vi "Diagnostics - Tool.vi"() -> ()   [LabVIEW 2015, in "Diagnostics Tool.lvlib"]
uses:
  Diagnostics Tool.lvlib
  Shared/Types/Command.ctl
  NationalInstruments.VeriStand.SystemStorage
  Shared/Types/Workspace.State.ctl
  Shared/Types/UI.Refs.ctl
  <vilib>/NI Veristand/Display Template Support/Display Template Support.llb/enum_Display Template Handler Minimal To Workspace.ctl
  Shared/Types/Workspace.SavedState.ctl
  <vilib>/NI Veristand/Execution/Workspace/WorkspaceAPI.ctl
  <vilib>/NI Veristand/Display Template Support/Display Template Support.llb/enum_Display Template Handler Minimal To Widget Msg.ctl
  <vilib>/NI Veristand/Execution/Workspace/SystemStateRegEventRef.ctl
  <vilib>/NI Veristand/Execution/Workspace/Target State Info.ctl
  <vilib>/NI Veristand/Execution/Workspace/Target State.ctl
  <vilib>/NI Veristand/Execution/Workspace/SystemStateEventRef.ctl
  Shared/Types/Protocol.ctl
  Shared/Types/Command.ReadDTC.ctl
  Shared/SubVIs/Constants.vi
  <vilib>/NI Veristand/Execution/Workspace/NI VeriStand - Get Multiple Channel Values.vi
  <vilib>/NI Veristand/Execution/Workspace/NI VeriStand - Set Multiple Channel Values.vi
  Shared/Diagnostics Addon Shared.lvlib
  <vilib>/NI Veristand/Execution/Workspace/NI_VS Workspace ExecutionAPI.lvlib
  Automation API/Diagnostics Host Automation API.lvlib
  NationalInstruments.VeriStand.ClientAPI
panel:
  out "Control Name":string
  in  "Tab Control":enum32{"Cmd", "Raw (TCP)", "Read DTCs (TCP)"}(tab)
  in  "Send":bool
  out "Data Length":i64
  out "VeriStand Error":i64 format="%.0x"
  out "Error Byte":i64 format="%.0x"
  out "Success?":bool
  in  "MetaData1":i64 format="%.0x"
  in  "MetaData2":i64 format="%.0x"
  in  "MetaData3":i64 format="%.0x"
  in  "MetaData4":i64 format="%.0x"
  in  "Cmd":T1
  in  "Clear":bool
  out "VeriStand Error":errorcluster
  out "Error Byte":u8 format="%.0x"
  in  "Response Required?":bool
  in  "Send Raw":bool
  out "Raw Resp":u8[](array[numeric]) format="%.0x"
  in  "Raw Cmd":u8[](array[numeric]) format="%.0x"
  in  "Extension":u32 format="%.0x"
  in  "Mask":u32 format="%.0x"
  in  "Mode":u32 format="%.0x"
  in  "Hex":bool
  in  "DTCs":i32(listbox)
  in  "Read DTCs":bool
  in  "NIVS.Gateway IP Address":string
  in  "NIVS.System Definition Root":refnum<k24>
  in  "NIVS.Workspace Event":refnum<event-registration>
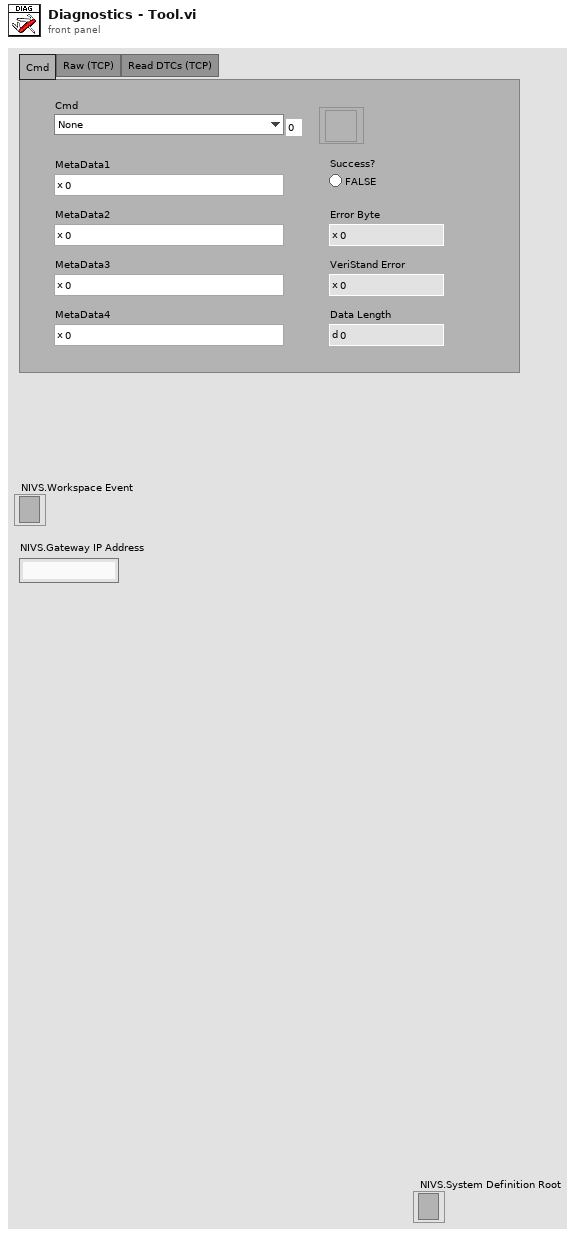
[diagram p1: front panel]
types:
  T1 = typedef "Diagnostics Addon Shared.lvlib/Command.ctl" = enum8{"None", "EnableDiagnosticSession", "DisableDiagnosticSession", "ReadDataIdentifiers", "ReadDataIdentifier", "WriteDataIndentifier", "ReadPIDsOnDemand", "ReadPIDOnDemand", "WriteCPID", "WriteMemory", "ReadMemory", "ReadDTCs", "ClearDTCs", "ControlDTC", "ForceTesterPresent", "DisableNormalCommunication", "ReturnToNormalMode", "InputOutputControl", "StartRoutine", "RequestRoutineStatus", "StopRoutine", "ECUReset", "UnlockECU", "ClearSuccessBit", "ConfigureandStartPIDs", "StopPIDs", "StartDTCs", "EnableChangeDTCCount", "DisableChangeDTCCount", "ReadFailureRecordParameters", "PassThru Channel Based", "EnableRepeatingTesterPresent", "DisableRepeatingTesterPresent"}
  T2 = typedef "Diagnostics Addon Shared.lvlib/Workspace.State.ctl" = cluster{"UI.Refs":T3, "Data.PreviousValues":dbl[], "Data.Read":string[], "CachedData.UserEvent":refnum<user-event>, "CachedData":T4, "Workspace.Connected?":bool, "NIVS.SysDef":refnum<k24>, "NIVS.WorkspaceManager":T5, "NIVS.UserEventRefs":cluster{"Event Registration Refnum":refnum<event-registration>, "SystemChangeEventRef":T6, "NIVS.Workspace Event":refnum<event-registration>}, "NIVS.SystemStateRefs":T7, "NIVS.LaunchRef":refnum<user-event>, "Data.PendingChange?":bool, "Data.Write":string[], "Diagnostic Protocol":T8, "Channels.Found":bool}
  T3 = typedef "Diagnostics Addon Shared.lvlib/UI.Refs.ctl" = cluster{"Cmd":refnum<vi>, "MetaData1":refnum<vi>, "MetaData2":refnum<vi>, "MetaData3":refnum<vi>, "MetaData4":refnum<vi>, "Success?":refnum<vi>, "ErrorByte":refnum<vi>, "VeriStandError":refnum<vi>, "DataLength":refnum<vi>}
  T4 = typedef "Diagnostics Addon Shared.lvlib/Workspace.SavedState.ctl" = cluster{"CD Path":string, "CD IP":string}
  T5 = typedef "NI_VS Workspace ExecutionAPI.lvlib/WorkspaceAPI.ctl" = refnum<k24>
  T6 = typedef "NI_VS Workspace ExecutionAPI.lvlib/SystemStateRegEventRef.ctl" = refnum<event-registration>
  T7 = typedef "NI_VS Workspace ExecutionAPI.lvlib/SystemStateEventRef.ctl" = cluster{"CustDatRef":refnum<user-event>, "EvtRef":refnum<k27>, "Target State User Event":refnum<user-event>}
  T8 = typedef "Diagnostics Addon Shared.lvlib/Protocol.ctl" = enum16{"GMLAN", "KWP-2000", "UDS", "User-Defined"}
  T9 = typedef "enum_Display Template Handler Minimal To Workspace.ctl" = cluster{"Operation":enum16{"SetCustomData", "DeleteItem"}, "Data":variant}
  T10 = typedef "Diagnostics Addon Shared.lvlib/Command.ReadDTC.ctl" = cluster{"Extension":u32, "Mask":u32, "Mode":u32}
  T11 = cluster{"Event Registration Refnum":refnum<event-registration>, "SystemChangeEventRef":T6, "NIVS.Workspace Event":refnum<event-registration>}
  T12 = typedef "NI_VS Workspace ExecutionAPI.lvlib/SystemState.ctl" = u8
  T13 = typedef "enum_Display Template Handler Minimal To Widget Msg.ctl" = enum16{"Stop", "LaunchConfigDialog"}
  T14 = typedef "stm_TCP Connection Info.ctl" = cluster{"connection ID":refnum<k5>, "Meta data":T15[]}
  T15 = typedef "stm_MetaDataElement.ctl" = string
  T16 = cluster{"resp":u8[], "error code":u8, "error out":errorcluster}
  T17 = typedef "Diagnostics Addon Shared.lvlib/DTC.Info.ctl" = cluster{"Timestamp":dbl, "DTC":dbl, "Status":dbl, "Add Data":dbl}
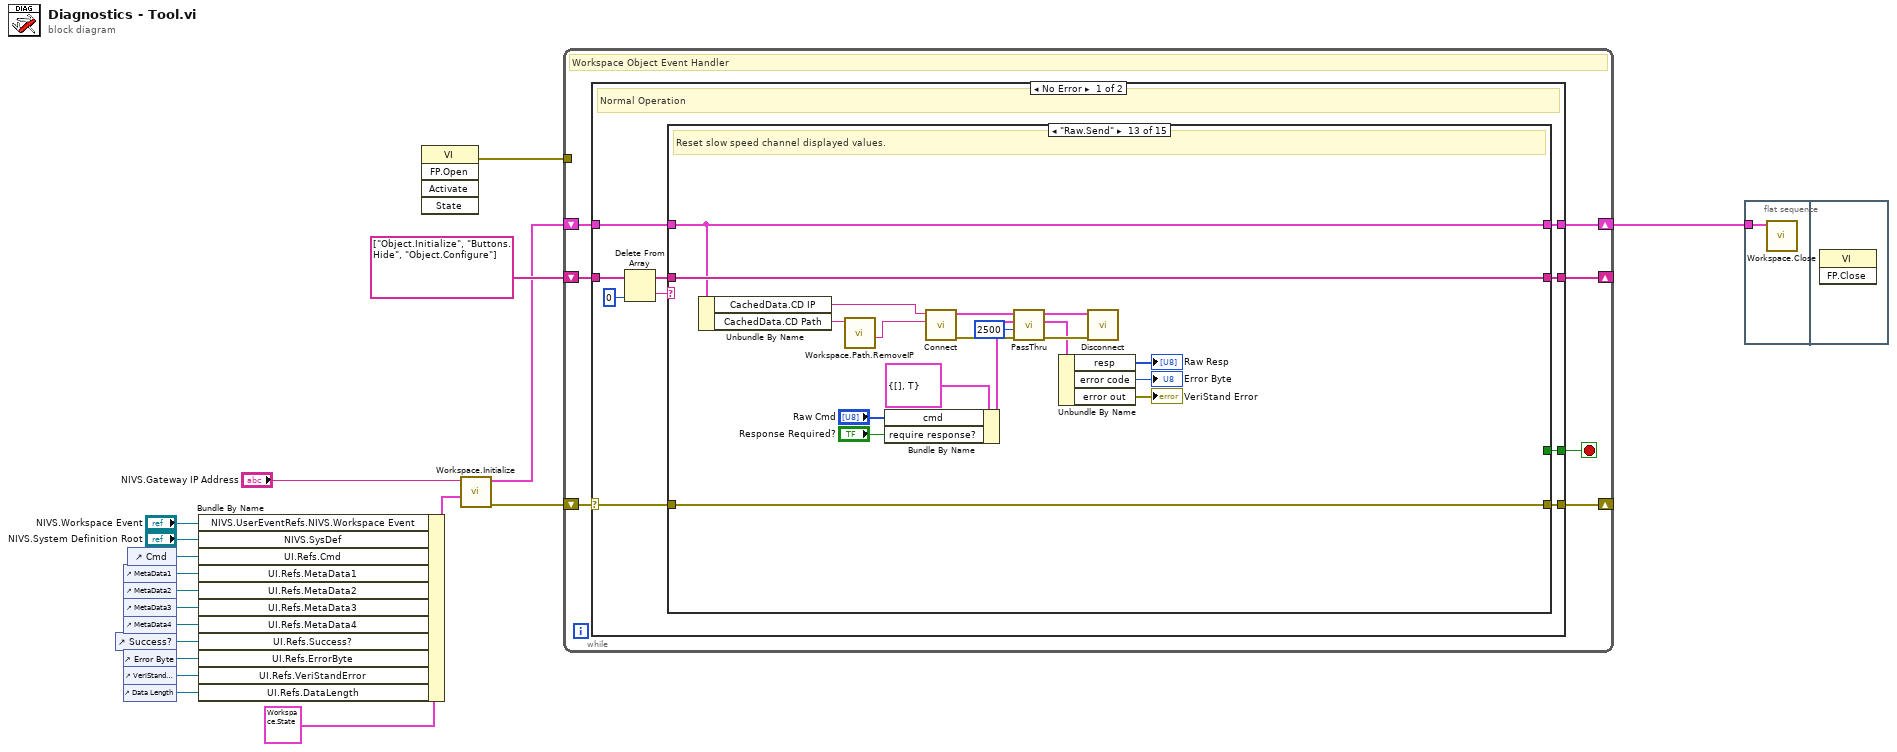
[diagram p0: block diagram]
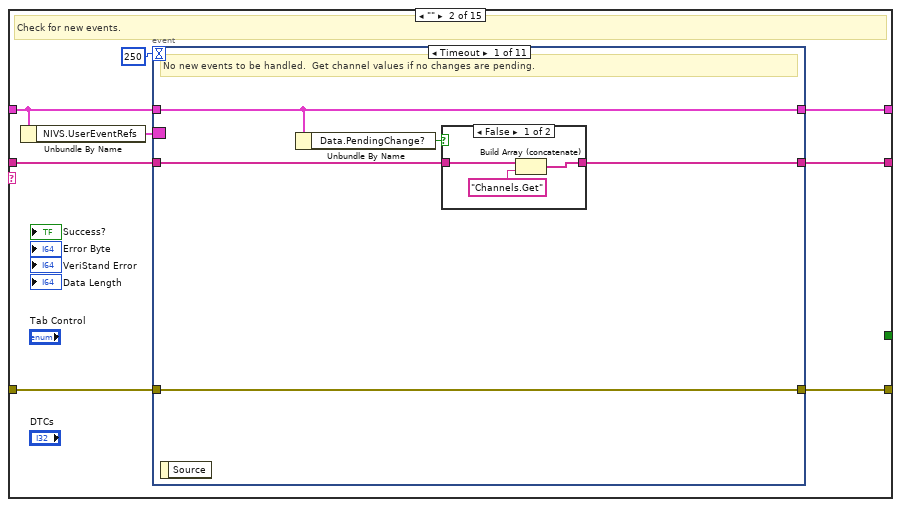
[diagram p3: hidden frame]
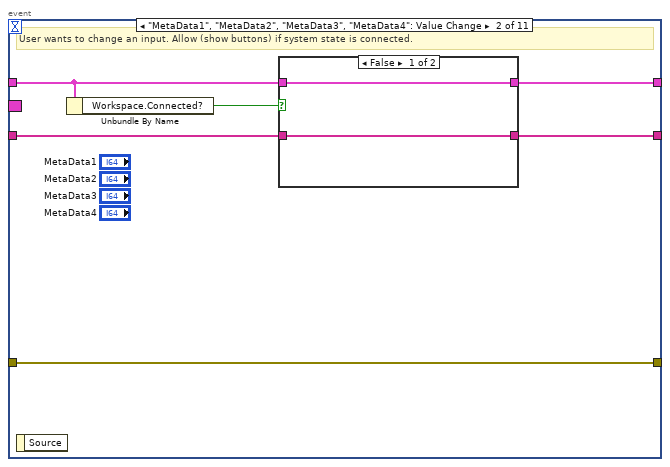
[diagram p5: hidden frame]
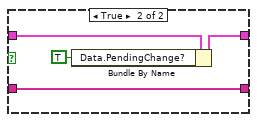
[diagram p6: hidden frame]
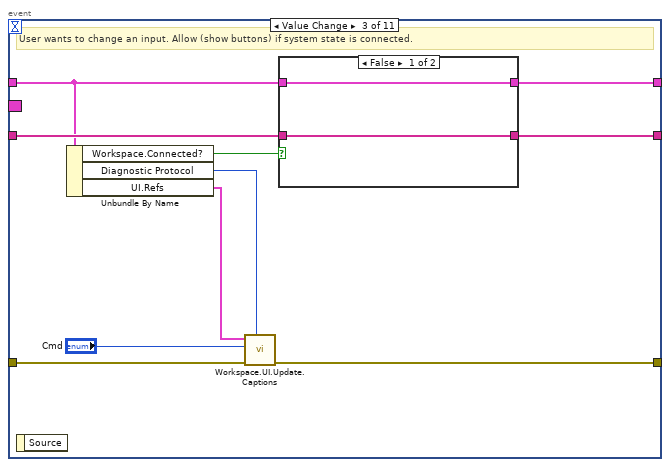
[diagram p7: hidden frame]
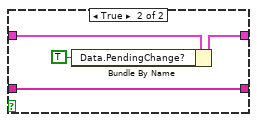
[diagram p8: hidden frame]
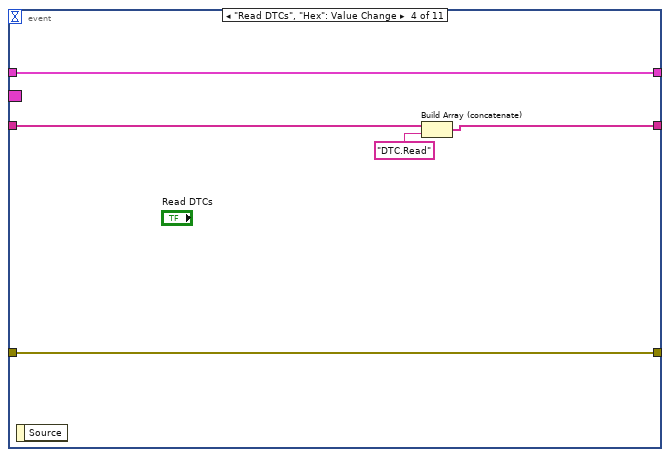
[diagram p9: hidden frame]
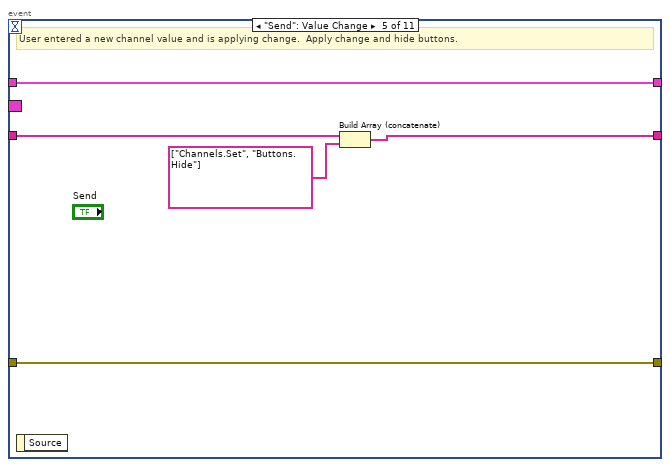
[diagram p10: hidden frame]
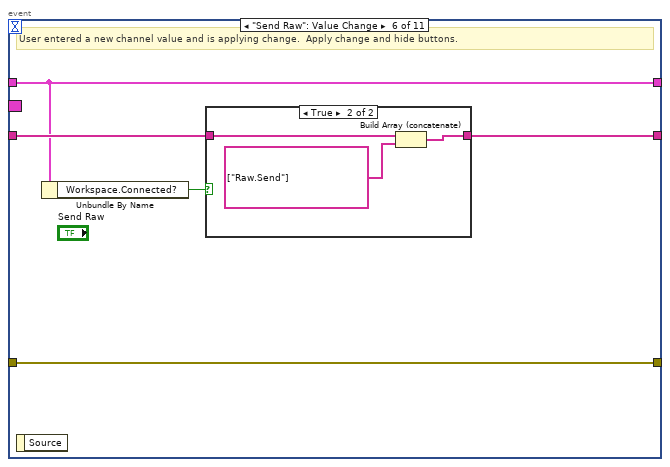
[diagram p11: hidden frame]
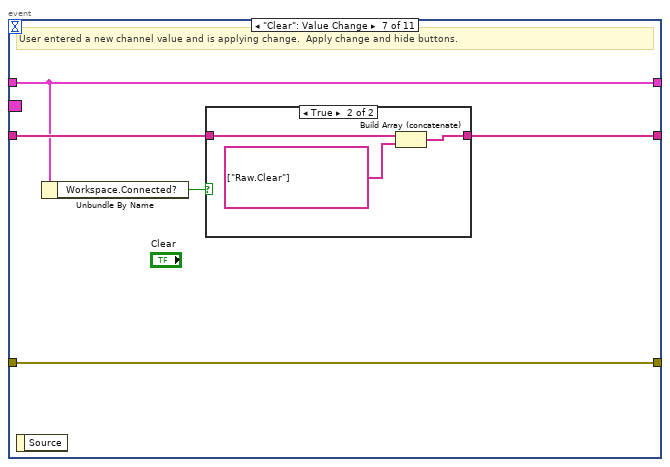
[diagram p13: hidden frame]
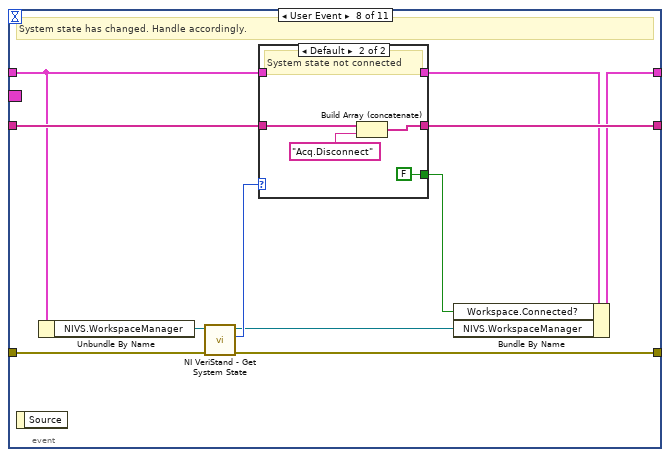
[diagram p15: hidden frame]
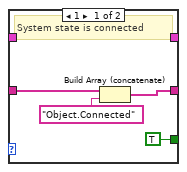
[diagram p16: hidden frame]
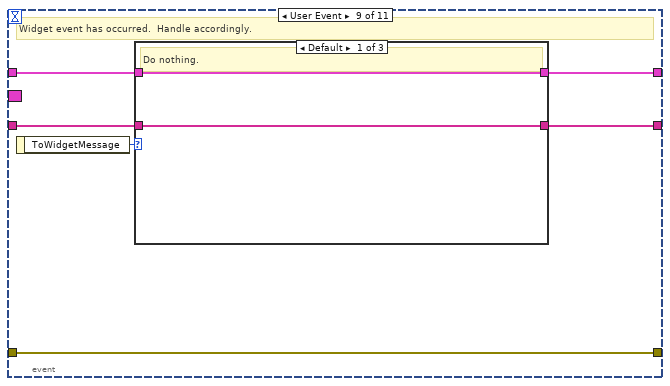
[diagram p17: hidden frame]
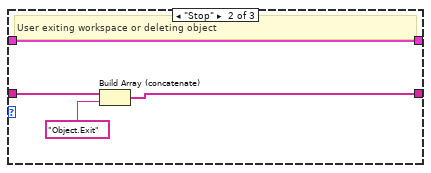
[diagram p18: hidden frame]
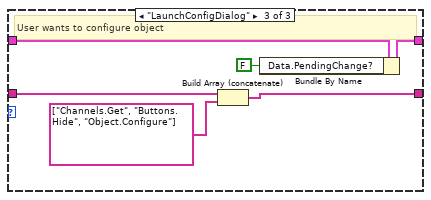
[diagram p19: hidden frame]
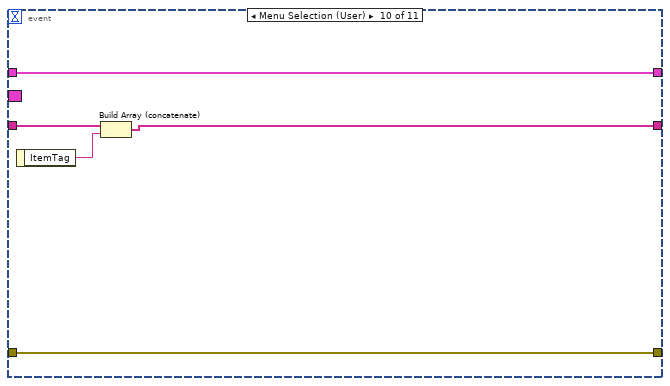
[diagram p20: hidden frame]
diagram:
  n1 = control-ref of="Success?"() -> (w4:refnum<vi>)
  n2 = control-ref of="MetaData1"() -> (w8:refnum<vi>)
  n3 = control-ref of="MetaData2"() -> (w7:refnum<vi>)
  n4 = control-ref of="MetaData3"() -> (w6:refnum<vi>)
  n5 = control-ref of="MetaData4"() -> (w5:refnum<vi>)
  n6 = control-ref of="Error Byte"() -> (w3:refnum<vi>)
  n7 = control-ref of="VeriStand Error"() -> (w2:refnum<vi>)
  n8 = control-ref of="Data Length"() -> (w1:refnum<vi>)
  n9 = control-ref of="Cmd"() -> (w9:refnum<vi>)
  n10 = Bundle By Name(cluster=T2 {"UI.Refs"={"Cmd"=refnum, "MetaData1"=refnum, "MetaData2"=refnum, "MetaData3"=refnum, "MetaData4"=refnum, "Success?"=refnum, "ErrorByte"=refnum, "VeriStandError"=refnum, "DataLength"=refnum}, "Data.PreviousValues"=[], "Data.Read"=[], "CachedData.UserEvent"=refnum, "CachedData"={"CD Path"="", "CD IP"=""}, "Workspace.Connected?"=FALSE, "NIVS.SysDef"=refnum, "NIVS.WorkspaceManager"=refnum, "NIVS.UserEventRefs"={"Event Registration Refnum"=refnum, "SystemChangeEventRef"=refnum, "NIVS.Workspace Event"=refnum}, "NIVS.SystemStateRefs"={"CustDatRef"=refnum, "EvtRef"=refnum, "Target State User Event"=refnum}, "NIVS.LaunchRef"=refnum, "Data.PendingChange?"=FALSE, "Data.Write"=[], "Diagnostic Protocol"=enum."GMLAN", "Channels.Found"=FALSE}, "NIVS.UserEventRefs.NIVS.Workspace Event"="NIVS.Workspace Event", "NIVS.SysDef"="NIVS.System Definition Root", "UI.Refs.Cmd"=w9, "UI.Refs.MetaData1"=w8, "UI.Refs.MetaData2"=w7, "UI.Refs.MetaData3"=w6, "UI.Refs.MetaData4"=w5, "UI.Refs.Success?"=w4, "UI.Refs.ErrorByte"=w3, "UI.Refs.VeriStandError"=w2, "UI.Refs.DataLength"=w1) -> (w18:T2)
  n11 = invoke class="VI" method="FP.Open"() -> (error out=w11:errorcluster)  [unwired: 5 in, 4 out]
  n12 = call "Workspace.Initialize.vi"("State Variables in"=w18, "NIVS.Gateway IP Address"="NIVS.Gateway IP Address") -> ("error out"=w14:errorcluster, "State Variables out"=w12:T2)  [unwired: 8 in]
  n13 = while {
    shift-right: [w24] -> _
    shift-left: string[] ["Object.Initialize", "Buttons.Hide", "Object.Configure"] -> [w25]
    shift-right: [w22] -> w10
    shift-left: w12 -> [w21]
    shift-right: [w23] -> _
    shift-left: w14 -> [w20]
    tunnel: w11 -> [_]
    stop <- w26 stop-if-true
    # "Workspace Object Event Handler"
    n14 = case shown="No Error" w20 {
      selector: w20 -> [w27 w385]
      tunnel: [w36 _] -> w26
      tunnel: w25 -> [w34 w392]
      tunnel: [w31 w392] -> w24
      tunnel: [w30 w383] -> w23
      tunnel: [w29 w391] -> w22
      tunnel: w21 -> [w28 w391]
      frame No Error {
        # "Normal Operation"
        n15 = Delete From Array(array=w34, index=0) -> (deleted portion=w33:string, array with subset deleted=w32:string[])  [unwired: 1 in]
        n16 = case shown="\"Raw.Send\"" w33 {
          tunnel: [_ _ _ _ _ TRUE _ _ _ _ _ _ _ _ _] -> w36
          tunnel: [w39 w46 w182 w199 w230 w246 w253 w256 w259 w268 w301 w314 w333 w337 w358] -> w31
          tunnel: w27 -> [w38 w44 w183 w205 w227 w243 w252 w254 w257 w266 w300 w313 w332 w336 w346]
          tunnel: w32 -> [w39 w45 w169 w198 w230 w246 w253 w256 w259 w268 w301 w314 w333 w337 w358]
          tunnel: w28 -> [w37 w40 w174 w203 w232 w244 w249 w255 w258 w260 w298 w312 w329 w335 w357]
          tunnel: [w38 w43 w164 w205 w217 w243 w252 w254 w257 w265 w299 w313 w332 w336 w345] -> w30
          tunnel: [w37 w42 w177 w202 w231 w244 w249 w255 w258 w264 w297 w312 w329 w335 w357] -> w29
          frame Default {
            # "Do nothing."
          }
          frame "" {
            # "Check for new events."
            n17 = Unbundle By Name(w40) -> ("NIVS.UserEventRefs"=w41:T11)
            n18 = event shown="[0] Timeout" {
              selector: w41 -> [_ _ _ _ _ _ _ _ _ _ _]
              dyn-events: _ -> [_ _ _ _ _ _ _ _ _ _ _]
              timeout: 250 -> [_ _ _ _ _ _ _ _ _ _ _]
              tunnel: [w50 w60 w76 w85 w90 w97 w106 w119 w138 w152 w159] -> w46
              tunnel: w45 -> [w51 w61 w77 w86 w91 w98 w107 w120 w137 w153 w160]
              tunnel: w44 -> [w52 w57 w73 w89 w94 w99 w108 w123 w136 w156 w162]
              tunnel: [w52 w57 w72 w89 w94 w99 w108 w122 w136 w156 w162] -> w43
              tunnel: [w49 w62 w78 w88 w93 w96 w105 w118 w134 w155 w161] -> w42
              tunnel: w40 -> [w49 w59 w75 w88 w93 w96 w105 w115 w135 w155 w161]
              event Timeout {
                # "No new events to be handled.  Get channel values if no changes are pending."
                n19 = event-data() -> ()  [unwired: 2 out]
                n20 = Unbundle By Name(w49) -> ("Data.PendingChange?"=w48:bool)
                n21 = case shown="False" w48 {
                  tunnel: w51 -> [w54 w56]
                  tunnel: [w53 w56] -> w50
                  frame False {
                    n22 = Build Array (concatenate)(w54, "Channels.Get") -> (w53:string[])
                  }
                  frame True {
                  }
                }
              }
              event "MetaData1", "MetaData2", "MetaData3", "MetaData4": Value Change {
                # "User wants to change an input. Allow (show buttons) if system state is connected."
                n23 = event-data() -> ()  [unwired: 2 out]
                n24 = Unbundle By Name(w59) -> ("Workspace.Connected?"=w58:bool)
                n25 = case shown="False" w58 {
                  tunnel: w59 -> [w63 w67]
                  tunnel: [w63 w66] -> w62
                  tunnel: w61 -> [w64 w65]
                  tunnel: [w64 w65] -> w60
                  frame False {
                  }
                  frame True {
                    n26 = Bundle By Name(cluster=w67, "Data.PendingChange?"=TRUE ("Pending Change?")) -> (w66:T2)
                  }
                }
              }
              event Value Change {
                # "User wants to change an input. Allow (show buttons) if system state is connected."
                n27 = event-data() -> ()  [unwired: 2 out]
                n28 = Unbundle By Name(w75) -> ("Workspace.Connected?"=w74:bool, "Diagnostic Protocol"=w69:T8, "UI.Refs"=w71:T3)
                n29 = call "Workspace.UI.Update.Captions.vi"("Diagnostic Protocol"=w69, "error in (no error)"=w73, "Cmd"="Cmd", "UI.Refs"=w71) -> ("error out"=w72:errorcluster)  [unwired: 7 in]
                n30 = case shown="False" w74 {
                  tunnel: w75 -> [w79 w83]
                  tunnel: [w79 w82] -> w78
                  tunnel: w77 -> [w80 w81]
                  tunnel: [w80 w81] -> w76
                  frame False {
                  }
                  frame True {
                    n31 = Bundle By Name(cluster=w83, "Data.PendingChange?"=TRUE ("Pending Change?")) -> (w82:T2)
                  }
                }
              }
              event "Read DTCs", "Hex": Value Change {
                n32 = event-data() -> ()  [unwired: 2 out]
                n33 = Build Array (concatenate)(w86, "DTC.Read") -> (w85:string[])
              }
              event "Send": Value Change {
                # "User entered a new channel value and is applying change.  Apply change and hide buttons."
                n34 = event-data() -> ()  [unwired: 2 out]
                n35 = Build Array (concatenate)(w91, string[] ["Channels.Set", "Buttons.Hide"]) -> (w90:string[])
              }
              event "Send Raw": Value Change {
                # "User entered a new channel value and is applying change.  Apply change and hide buttons."
                n36 = event-data() -> ()  [unwired: 2 out]
                n37 = Unbundle By Name(w96) -> ("Workspace.Connected?"=w95:bool)
                n38 = case shown="True" w95 {
                  tunnel: w98 -> [w100 w102]
                  tunnel: [w100 w101] -> w97
                  frame False {
                  }
                  frame True {
                    n39 = Build Array (concatenate)(w102, string[] ["Raw.Send"]) -> (w101:string[])
                  }
                }
              }
              event "Clear": Value Change {
                # "User entered a new channel value and is applying change.  Apply change and hide buttons."
                n40 = event-data() -> ()  [unwired: 2 out]
                n41 = Unbundle By Name(w105) -> ("Workspace.Connected?"=w104:bool)
                n42 = case shown="True" w104 {
                  tunnel: w107 -> [w109 w111]
                  tunnel: [w109 w110] -> w106
                  frame False {
                  }
                  frame True {
                    n43 = Build Array (concatenate)(w111, string[] ["Raw.Clear"]) -> (w110:string[])
                  }
                }
              }
              event User Event {
                # "System state has changed. Handle accordingly."
                n44 = event-data() -> ()  [unwired: 2 out]
                n45 = Unbundle By Name(w115) -> ("NIVS.WorkspaceManager"=w114:T5)
                n46 = call <vilib>:"NI VeriStand - Get System State.vi"("error in (no error)"=w123, "WorkspaceManager in"=w114) -> ("error out"=w122:errorcluster, "System State"=w121:T12, "WorkspaceManager  out"=w113:T5)  [unwired: 5 in, 2 out]
                n47 = case shown="Default" w121 {
                  tunnel: w120 -> [w128 w133]
                  tunnel: [w127 w132] -> w119
                  tunnel: [w125 w130] -> w117
                  tunnel: w115 -> [w125 w130]
                  tunnel: [TRUE FALSE] -> w116
                  frame 1 {
                    # "System state is connected"
                    n48 = Build Array (concatenate)(w128, "Object.Connected") -> (w127:string[])
                  }
                  frame Default {
                    # "System state not connected"
                    n49 = Build Array (concatenate)(w133, "Acq.Disconnect") -> (w132:string[])
                  }
                }
                n50 = Bundle By Name(cluster=w117, "Workspace.Connected?"=w116, "NIVS.WorkspaceManager"=w113) -> (w118:T2)
              }
              event User Event {
                # "Widget event has occurred.  Handle accordingly."
                n51 = event-data() -> ("ToWidgetMessage"=w139:T13)  [unwired: 1 out]
                n52 = case shown="Default" w139 {
                  tunnel: [w141 w144 w150] -> w138
                  tunnel: w137 -> [w141 w145 w151]
                  tunnel: w135 -> [w140 w142 w147]
                  tunnel: [w140 w142 w146] -> w134
                  frame Default {
                    # "Do nothing."
                  }
                  frame "Stop" {
                    # "User exiting workspace or deleting object"
                    n53 = Build Array (concatenate)(w145, "Object.Exit") -> (w144:string[])
                  }
                  frame "LaunchConfigDialog" {
                    # "User wants to configure object"
                    n54 = Build Array (concatenate)(w151, string[] ["Channels.Get", "Buttons.Hide", "Object.Configure"]) -> (w150:string[])
                    n55 = Bundle By Name(cluster=w147, "Data.PendingChange?"=FALSE ("Pending Change?")) -> (w146:T2)
                  }
                }
              }
              event Menu Selection (User) {
                n56 = event-data() -> ("ItemTag"=w154:string)  [unwired: 1 out]
                n57 = Build Array (concatenate)(w153, w154) -> (w152:string[])
              }
              event Panel Close? {
                n58 = event-data() -> ()  [unwired: 5 out]
                n59 = Build Array (concatenate)(w160, "Object.Exit") -> (w159:string[])
                n60 = event-data("Discard?"=TRUE) -> ()  [unwired: 1 in, 1 out]
              }
            }
          }
          frame "Object.Initialize" {
            # "Initialize the workspace Object state variables and UI"
            n61 = Unbundle By Name(w174) -> ("CachedData.CD Path"=w166:string, "NIVS.WorkspaceManager"=w173:T5)
            n62 = Build Array (concatenate)(w169, "UI.ResetChannels") -> (w168:string[])
            n63 = call "Workspace.Path.RemoveIP.vi"("CD Path"=w166) -> ("Path"=w171:string)  [unwired: 9 in, 1 out]
            n64 = call <vilib>:"NI VeriStand - Get System State.vi"("error in (no error)"=w183, "WorkspaceManager in"=w173) -> ("error out"=w165:errorcluster, "System State"=w184:T12, "WorkspaceManager  out"=w172:T5)  [unwired: 5 in, 2 out]
            n65 = case shown="1" w184 {
              tunnel: w168 -> [w189 w194]
              tunnel: [w188 w194] -> w182
              tunnel: [TRUE FALSE] -> w176
              tunnel: w166 -> [w186 _]
              frame 1 {
                n66 = Empty String/Path?(string/path=w186) -> (empty?=w185:bool)
                n67 = case shown="True" w185 {
                  tunnel: w189 -> [w192 w193]
                  tunnel: [w191 w193] -> w188
                  frame False {
                    n68 = Build Array (concatenate)(w192, "Object.Connected") -> (w191:string[])
                  }
                  frame True {
                  }
                }
              }
              frame Default {
              }
            }
            n69 = Reverse String(1:w171) -> (0:w181:string)
            n70 = Match Pattern(string=w181, regular expression="/") -> (before substring=w178:string)  [unwired: 1 in, 3 out]
            n71 = Reverse String(1:w178) -> (0:→"Control Name":string)
            n72 = property on="DTCs" class="MCListbox (strict)"(error in=w165, "ItemNames"=string[][] [] ("Item Names")) -> (error out=w164:errorcluster)  [unwired: 1 in, 1 out]
            n73 = local write "Tab Control"(0) -> ()
            n74 = Bundle By Name(cluster=w174, "Workspace.Connected?"=w176, "Data.PendingChange?"=FALSE ("Pending Change?"), "NIVS.WorkspaceManager"=w172) -> (w177:T2)
          }
          frame "Object.Configure" {
            # "Allow the user to select a control object to display"
            n75 = Unbundle By Name(w203) -> ("NIVS.SysDef"=w197:refnum<k24>, "CachedData.CD Path"=w204:string)
            n76 = call "Workspace.Select.Dialog.vi"("CD Path"=w204, "NIVS.System Definition Root"=w197) -> ("Cancelled?"=w201:bool, "IP Address"=w196:string, "Custom Device Path Out"=w200:string)  [unwired: 7 in]
            n77 = case shown="False" w201 {
              tunnel: w203 -> [w212 w213]
              tunnel: [w211 w213] -> w202
              tunnel: w200 -> [w210 _]
              tunnel: [w208 w214] -> w199
              tunnel: w198 -> [w209 w214]
              tunnel: w196 -> [w206 _]
              frame False {
                # "Queue up required states and cache new controller path"
                n78 = Bundle By Name(cluster=w212, "CachedData.CD Path"=w210, "CachedData.CD IP"=w206) -> (w211:T2)
                n79 = Build Array (concatenate)(w209, string[] ["Cache.Update", "Object.Initialize"]) -> (w208:string[])
              }
              frame True {
                # "User canceled"
              }
            }
          }
          frame "Object.Connected" {
            # "System state is Connected. Get path to required channels and start UDP acquisition if channels found."
            n80 = Unbundle By Name(w232) -> ("CachedData.CD Path"=w226:string, "NIVS.SysDef"=w224:refnum<k24>, "UI.Refs.Cmd"=w216:refnum<vi>)
            n81 = call "Workspace.Path.RemoveIP.vi"("CD Path"=w226) -> ("Path"=w225:string)  [unwired: 9 in, 1 out]
            n82 = call "Workspace.CAN.Protocol.Get.vi"("error in (no error)"=w227, "Path"=w225, "NIVS.SysDef Ref"=w224) -> ("error out"=w218:errorcluster, "Diagnostic Protocol"=w215:T8)  [unwired: 7 in]
            n83 = call "Workspace.Channels.Create.vi"("CD Path"=w226) -> ("Read Channels"=w229:string[], "Write Channels"=w228:string[])  [unwired: 9 in]
            n84 = case shown="\"User-Defined\"" w215 {
              tunnel: [w238 w240 w242] -> w219
              tunnel: [bool[] [TRUE, TRUE, TRUE] bool[] [TRUE, TRUE, TRUE] bool[] [TRUE, TRUE, FALSE]] -> w222
              frame "GMLAN" {
                w238 = T1[] [enum."ECUReset", enum."WriteMemory", enum."ReadMemory", enum."InputOutputControl", enum."StartRoutine", enum."RequestRoutineStatus", enum."StopRoutine", enum."ControlDTC", enum."ReadDTCs", enum."WriteDataIndentifier"] items=["None", "EnableDiagnosticSession", "DisableDiagnosticSession", "ReadDataIdentifiers", "ReadDataIdentifier", "WriteDataIndentifier", "ReadPIDsOnDemand", "ReadPIDOnDemand", "WriteCPID", "WriteMemory", "ReadMemory", "ReadDTCs", "ClearDTCs", "ControlDTC", "ForceTesterPresent", "DisableNormalCommunication", "ReturnToNormalMode", "InputOutputControl", "StartRoutine", "RequestRoutineStatus", "StopRoutine", "ECUReset", "UnlockECU", "ClearSuccessBit", "ConfigureandStartPIDs", "StopPIDs", "StartDTCs", "EnableChangeDTCCount", "DisableChangeDTCCount", "ReadFailureRecordParameters", "PassThru Channel Based", "EnableRepeatingTesterPresent", "DisableRepeatingTesterPresent"] ("Disabled Items []")
              }
              frame "KWP-2000", "UDS" {
                w240 = T1[] [enum."EnableChangeDTCCount", enum."DisableChangeDTCCount", enum."StartDTCs", enum."ReadFailureRecordParameters", enum."ConfigureandStartPIDs", enum."StopPIDs", enum."WriteCPID", enum."ReadPIDsOnDemand", enum."ReadPIDOnDemand"] items=["None", "EnableDiagnosticSession", "DisableDiagnosticSession", "ReadDataIdentifiers", "ReadDataIdentifier", "WriteDataIndentifier", "ReadPIDsOnDemand", "ReadPIDOnDemand", "WriteCPID", "WriteMemory", "ReadMemory", "ReadDTCs", "ClearDTCs", "ControlDTC", "ForceTesterPresent", "DisableNormalCommunication", "ReturnToNormalMode", "InputOutputControl", "StartRoutine", "RequestRoutineStatus", "StopRoutine", "ECUReset", "UnlockECU", "ClearSuccessBit", "ConfigureandStartPIDs", "StopPIDs", "StartDTCs", "EnableChangeDTCCount", "DisableChangeDTCCount", "ReadFailureRecordParameters", "PassThru Channel Based", "EnableRepeatingTesterPresent", "DisableRepeatingTesterPresent"] ("Disabled Items []")
              }
              frame "User-Defined" {
                w242 = T1[] [enum."EnableDiagnosticSession", enum."DisableDiagnosticSession", enum."ReadDataIdentifiers", enum."ReadDataIdentifier", enum."WriteDataIndentifier", enum."ReadPIDsOnDemand", enum."ReadPIDOnDemand", enum."WriteCPID", enum."WriteMemory", enum."ReadMemory", enum."ReadDTCs", enum."ClearDTCs", enum."ControlDTC", enum."ForceTesterPresent", enum."DisableNormalCommunication", enum."ReturnToNormalMode", enum."InputOutputControl", enum."StartRoutine", enum."RequestRoutineStatus", enum."StopRoutine", enum."ECUReset", enum."UnlockECU", enum."ConfigureandStartPIDs", enum."StopPIDs", enum."StartDTCs", enum."EnableChangeDTCCount", enum."DisableChangeDTCCount", enum."ReadFailureRecordParameters"] items=["None", "EnableDiagnosticSession", "DisableDiagnosticSession", "ReadDataIdentifiers", "ReadDataIdentifier", "WriteDataIndentifier", "ReadPIDsOnDemand", "ReadPIDOnDemand", "WriteCPID", "WriteMemory", "ReadMemory", "ReadDTCs", "ClearDTCs", "ControlDTC", "ForceTesterPresent", "DisableNormalCommunication", "ReturnToNormalMode", "InputOutputControl", "StartRoutine", "RequestRoutineStatus", "StopRoutine", "ECUReset", "UnlockECU", "ClearSuccessBit", "ConfigureandStartPIDs", "StopPIDs", "StartDTCs", "EnableChangeDTCCount", "DisableChangeDTCCount", "ReadFailureRecordParameters", "PassThru Channel Based", "EnableRepeatingTesterPresent", "DisableRepeatingTesterPresent"] ("Disabled Items []")
              }
            }
            n85 = Bundle By Name(cluster=w232, "Data.Write"=w228, "Data.Read"=w229, "Diagnostic Protocol"=w215) -> (w231:T2)
            n86 = property class="Enum (strict)"(reference=w216, error in=w218, "Disabled Items []"=w219) -> (error out=w220:errorcluster)  [unwired: 1 out]
            n87 = property on="Tab Control" class="TabCtl (strict)"(error in=w220) -> (error out=w223:errorcluster, "Pages"=w221:refnum<vi>[])  [unwired: 1 in, 1 out]
            n88 = for {
              tunnel: w221 -> [w236] mode=indexing
              tunnel: w222 -> [w235] mode=indexing
              shift-right: [w233] -> w217
              shift-left: w223 -> [w234]
              n89 = property class="Page"(reference=w236, error in=w234, "PageVis"=w235) -> (error out=w233:errorcluster)  [unwired: 1 out]
            }
          }
          frame "Object.Exit" {
            # "Stop current loop.  Queue Stop Acq and Exit to UDP loop."
          }
          frame "Cache.Update" {
            # "Cache any data needing to be permenantly stored with the workspace object."
            n90 = Unbundle By Name(w249) -> ("CachedData.UserEvent"=w247:refnum<user-event>, "CachedData"=w248:T4)
            n91 = Bundle By Name(cluster=T9 {"Operation"=enum."SetCustomData", "Data"=variant} ("event data"), "Data"=w248) -> (w250:T9)
            n92 = Generate User Event(user event=w247, event data cluster=w250) -> ()  [unwired: 2 in, 2 out]
          }
          frame "Buttons.Hide" {
            # "Hide the apply and revert buttons from the user."
          }
          frame "Buttons.Show" {
            # "Show the apply and revert buttons to the user."
          }
          frame "Channels.Get" {
            # "Get the current slow speed channel values from VeriStand if no pending change, data paths are valid and system state is connected."
            n93 = Unbundle By Name(w260) -> ("Data.PendingChange?"=w261:bool, "Workspace.Connected?"=w267:bool, "NIVS.WorkspaceManager"=w263:T5, "Data.Read"=w262:string[])
            n94 = case shown="False" w261 {
              tunnel: w267 -> [w274 _]
              tunnel: w266 -> [w279 w289]
              tunnel: [w269 w289] -> w265
              tunnel: [w278 w290] -> w264
              tunnel: w263 -> [w277 _]
              tunnel: w262 -> [w275 _]
              tunnel: w260 -> [w272 w290]
              frame False {
                # "No pending data change.  Allow for a get."
                n95 = case shown="True" w274 {
                  tunnel: w279 -> [w282 w288]
                  tunnel: [w282 w287] -> w270
                  tunnel: w277 -> [w281 w286]
                  tunnel: [w281 w285] -> w276
                  tunnel: w275 -> [_ w284]
                  tunnel: [dbl[] [0.0, 0.0, 0.0] ("Values") w283] -> w273
                  frame False {
                    # "Do Nothing."
                  }
                  frame True {
                    # "Connected & paths valid"
                    n96 = call-poly <vilib>:"NI VeriStand - Get Channel Value.vi"("error in (no error)"=w288, "Channels"=w284, "WorkspaceManager in"=w286) -> ("error out"=w287:errorcluster, "Values"=w283:dbl[], "WorkspaceManager out"=w285:T5)  [unwired: 6 in]
                  }
                }
                n97 = Unbundle By Name(w272) -> ("UI.Refs"=w271:T3)
                n98 = call "Workspace.UI.Update.vi"("error in (no error)"=w270, "Values"=w273, "UI.Refs"=w271) -> ("error out"=w269:errorcluster)  [unwired: 8 in]
                n99 = Bundle By Name(cluster=w272, "NIVS.WorkspaceManager"=w276, "Data.PreviousValues"=w273) -> (w278:T2)
              }
              frame True {
                # "A change is pending.  Don't get channels as this would overwrite the pending change."
              }
            }
          }
          frame "Channels.Set" {
            # "Set Channels if data paths are valid and system state is connected and there is a change in the data value."
            n100 = Unbundle By Name(w298) -> ("Workspace.Connected?"=w294:bool, "NIVS.WorkspaceManager"=w293:T5, "Data.Write"=w291:string[], "UI.Refs"=w292:T3)
            n101 = case shown="True" w294 {
              tunnel: w300 -> [w303 w305]
              tunnel: [w303 w311] -> w299
              tunnel: w293 -> [w302 w310]
              tunnel: [w302 w309] -> w295
              tunnel: w291 -> [_ w308]
              tunnel: w292 -> [_ w306]
              frame False {
                # "Do nothing"
              }
              frame True {
                # "Connected & paths valid"
                n102 = call "Workspace.UI.Pull.vi"("error in (no error)"=w305, "UI.Refs"=w306) -> ("error out"=w304:errorcluster, "Values"=w307:dbl[])  [unwired: 8 in]
                n103 = call-poly <vilib>:"NI VeriStand - Set Channel Value.vi"("error in (no error)"=w304, "Values"=w307, "Channels"=w308, "WorkspaceManager in"=w310) -> ("error out"=w311:errorcluster, "WorkspaceManager out"=w309:T5)  [unwired: 6 in]
              }
            }
            n104 = Bundle By Name(cluster=w298, "Data.PendingChange?"=FALSE ("Pending Change?"), "NIVS.WorkspaceManager"=w295) -> (w297:T2)
          }
          frame "UI.ResetChannels" {
            # "Reset slow speed channel displayed values."
          }
          frame "Raw.Send" {
            # "Reset slow speed channel displayed values."
            n105 = Unbundle By Name(w329) -> ("CachedData.CD IP"=w317:string, "CachedData.CD Path"=w328:string)
            n106 = call "Workspace.Path.RemoveIP.vi"("CD Path"=w328) -> ("Name"=w316:string)  [unwired: 9 in, 1 out]
            n107 = Bundle By Name(cluster=cluster{"cmd":u8[], "require response?":bool} {"cmd"=[], "require response?"=TRUE} ("Cmd"), "cmd"="Raw Cmd", "require response?"="Response Required?") -> (w326:cluster{"cmd":u8[], "require response?":bool})
            n108 = call "Connect.vi"("Addon Name"=w316, "Address"=w317) -> ("error out"=w323:errorcluster, "Connection Info Out"=w330:T14)  [unwired: 8 in]
            n109 = call "PassThru.vi"("error in (no error)"=w323, "timeout ms (1000)"=2500, "Cmd"=w326, "Connection Info"=w330) -> ("error out"=w322:errorcluster, "Resp"=w321:T16, "Connection Info"=w331:T14)  [unwired: 5 in]
            n110 = Unbundle By Name(w321) -> ("resp"=→"Raw Resp":u8[], "error code"=→"Error Byte":u8, "error out"=→"VeriStand Error":errorcluster)
            n111 = call "Disconnect.vi"("error in"=w322, "Connection Info"=w331) -> ()  [unwired: 9 in, 1 out]
          }
          frame "Raw.Clear" {
            n112 = local write "Raw Cmd"(u8[] [] ("Cmd")) -> ()
          }
          frame "DTC.Read" {
            # "Reset slow speed channel displayed values."
            n113 = Unbundle By Name(w357) -> ("CachedData.CD IP"=w355:string, "CachedData.CD Path"=w356:string)
            n114 = call "Workspace.Path.RemoveIP.vi"("CD Path"=w356) -> ("Name"=w354:string)  [unwired: 9 in, 1 out]
            n115 = Bundle By Name(cluster=T10 {"Extension"=0, "Mask"=0, "Mode"=0} ("Options (KWP/UDS Only)"), "Extension"="Extension", "Mask"="Mask", "Mode"="Mode") -> (w343:T10)
            n116 = call "Connect.vi"("Addon Name"=w354, "Address"=w355) -> ("error out"=w352:errorcluster, "Connection Info Out"=w353:T14)  [unwired: 8 in]
            n117 = call "ReadDTCs.vi"("error in (no error)"=w352, "timeout ms (1000)"=2500, "Options (KWP/UDS Only)"=w343, "Connection Info"=w353) -> ("error out"=w351:errorcluster, "Active DTCs"=w349:T17[], "Connection Info"=w350:T14)  [unwired: 5 in]
            n118 = for {
              tunnel: w349 -> [w370] mode=indexing
              tunnel: "Hex" -> [w365]
              tunnel: [w359] -> w347 mode=indexing
              n119 = Unbundle By Name(w370) -> ("Timestamp"=w369:dbl, "DTC"=w368:dbl, "Status"=w367:dbl, "Add Data"=w366:dbl)
              n120 = To Time Stamp(1:w369) -> (0:w364:timestamp)
              n121 = case shown="False" w365 {
                tunnel: w368 -> [w376 w382]
                tunnel: w367 -> [w375 w381]
                tunnel: w366 -> [w374 w380]
                tunnel: [w373 w379] -> w360
                tunnel: [w372 w378] -> w361
                tunnel: [w371 w377] -> w362
                frame True {
                  n122 = Number To Hexadecimal String(2:w374) -> (0:w373:string)  [unwired: 1 in]
                  n123 = Number To Hexadecimal String(2:w375) -> (0:w372:string)  [unwired: 1 in]
                  n124 = Number To Hexadecimal String(2:w376) -> (0:w371:string)  [unwired: 1 in]
                }
                frame False {
                  n125 = Number To Decimal String(number=w380) -> (decimal integer string=w379:string)  [unwired: 1 in]
                  n126 = Number To Decimal String(number=w381) -> (decimal integer string=w378:string)  [unwired: 1 in]
                  n127 = Number To Decimal String(number=w382) -> (decimal integer string=w377:string)  [unwired: 1 in]
                }
              }
              n128 = Format Date/Time String(seconds (now)=w364) -> (date/time string=w363:string)  [unwired: 2 in]
              n129 = Build Array(w363, w362, w361, w360) -> (w359:string[])
            }
            n130 = call "Disconnect.vi"("error in"=w351, "Connection Info"=w350) -> ("error out"=w338:errorcluster)  [unwired: 9 in]
            n131 = call <vilib>:"Simple Error Handler.vi"("error in (no error)"=w338) -> ()  [unwired: 4 in, 5 out]
            n132 = property on="DTCs" class="MCListbox (strict)"(error in=w346, "ItemNames"=w347) -> (error out=w345:errorcluster)  [unwired: 1 in, 1 out]
          }
        }
      }
      frame Error {
        # "Handle Errors."
        n133 = Unbundle By Name(w385) -> ("code"=w389:i32)
        n134 = Equal?(x=-307654, y=w389) -> (x = y?=w387:bool)
        n135 = Select(t=errorcluster {"status"=FALSE, "code"=0, "source"=""}, s=w387, f=w385) -> (s? t:f=w384:errorcluster)
        n136 = call <vilib>:"Simple Error Handler.vi"("error in (no error)"=w384) -> ("error out"=w390:errorcluster)  [unwired: 4 in, 4 out]
        n137 = call <vilib>:"Clear Errors.vi"("error in (no error)"=w390) -> ("error out"=w383:errorcluster)  [unwired: 5 in, 1 out]
      }
    }
  }
  n138 = flat-sequence {
    tunnel: w10 -> [w393]
    frame #0 {
      n139 = call "Workspace.Close.vi"("State Variables in"=w393) -> ()  [unwired: 11 in]
    }
    frame #1 {
      n140 = invoke class="VI" method="FP.Close"() -> ()  [unwired: 3 in, 3 out]
    }
  }
